vi "Module - License.vi"(8 "Error In":errorcluster, 10 "License Filename":string="lcs_daq.bin", 11 "Product Name":string="VSys DAQ") -> (0 "Error Out":errorcluster, 1 "License Missing?":bool, 2 "Activate?":bool, 3 "License Info":T1={"Expired Time"="", "Computer ID"="", "Product Name"="", "Period"=0, "Activated Time"="", "License Level"=enum."Level 1", "License Type"=enum."Trial", "Log Time"=""}, 4 "Days left":i16)   [LabVIEW 2020]
doc: "This module handle the licensing part. It check the status of current license. If expired, msg will popup and ask user to activate a license or continue use as free user."
uses:
  Control/License File Parameter.ctl
  Control/State - Module License.ctl
  <vilib>/Utility/sysdir.llb/System Directory Type.ctl
panel:
  out "COMPUTER ID":string
  out "Expired?":bool
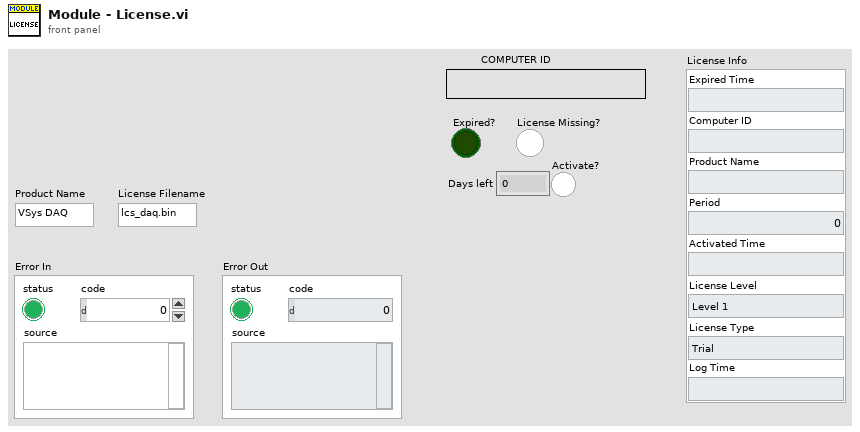
[diagram p1: front panel]
types:
  T1 = typedef "License File Parameter.ctl" = cluster{"Expired Time":string, "Computer ID":string, "Product Name":string, "Period":i16, "Activated Time":string, "License Level":enum16{"Level 1", "Level 2", "Level 3", "Level 4", "Level 5"}, "License Type":enum16{"Free", "Trial", "Subscription", "Perpetual"}, "Log Time":string}
  T2 = cluster{"T_Out":i32, "License File Param":T1, "Valid":bool, "License path":path, "Computer ID":string, "License Missing?":bool, "Path":path, "Activate?":bool, "Product Name":string, "License Filename":string, "Activation Path":path}
  T3 = typedef "State - Module License.ctl" = enum16{"Init", "Get Computer ID", "Check License File Exist?", "Copy License File", "Load License", "Check Log Time", "Check License Type", "Check License: Activated Date", "Update License: Activated Date", "Check License Period", "Update Log Time", "Check Computer ID", "Activate License: Expired", "Activate License: Trial", "Close"}
  T4 = enum16{"Free", "Trial", "Subscription", "Perpetual"}
  T5 = enum16{"Level 1", "Level 2", "Level 3", "Level 4", "Level 5"}
  T6 = enum32{"invalid app kind", "Development System", "Run Time System", "Student Edition", "Embedded LabVIEW", "Evaluation", "Custom"}
  T7 = typedef "System Directory Type.ctl" = i32
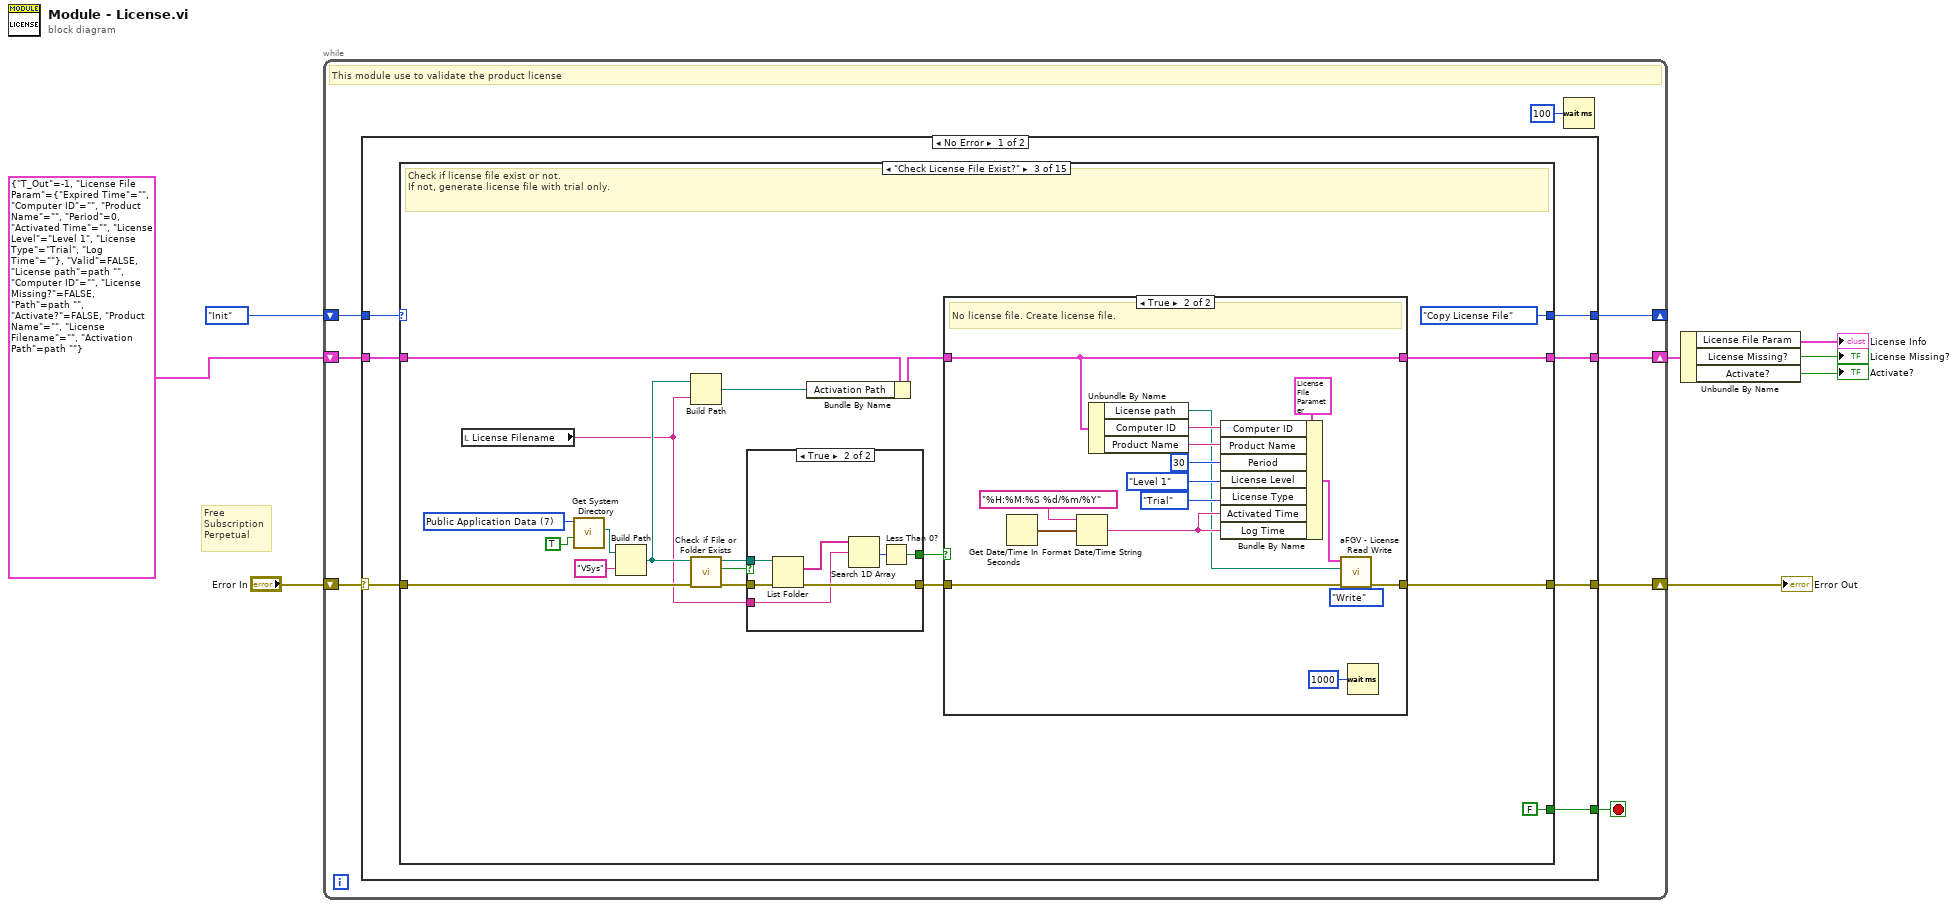
[diagram p0: block diagram]
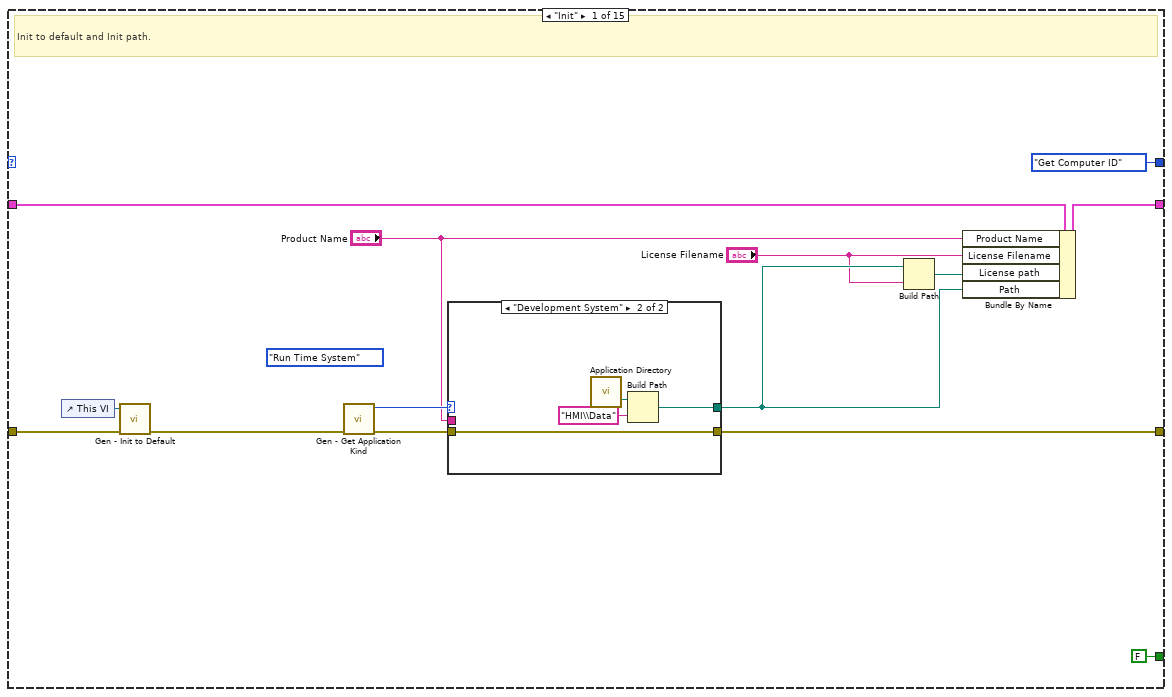
[diagram p2: hidden frame]
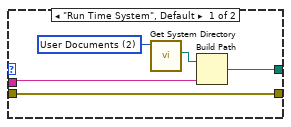
[diagram p3: hidden frame]
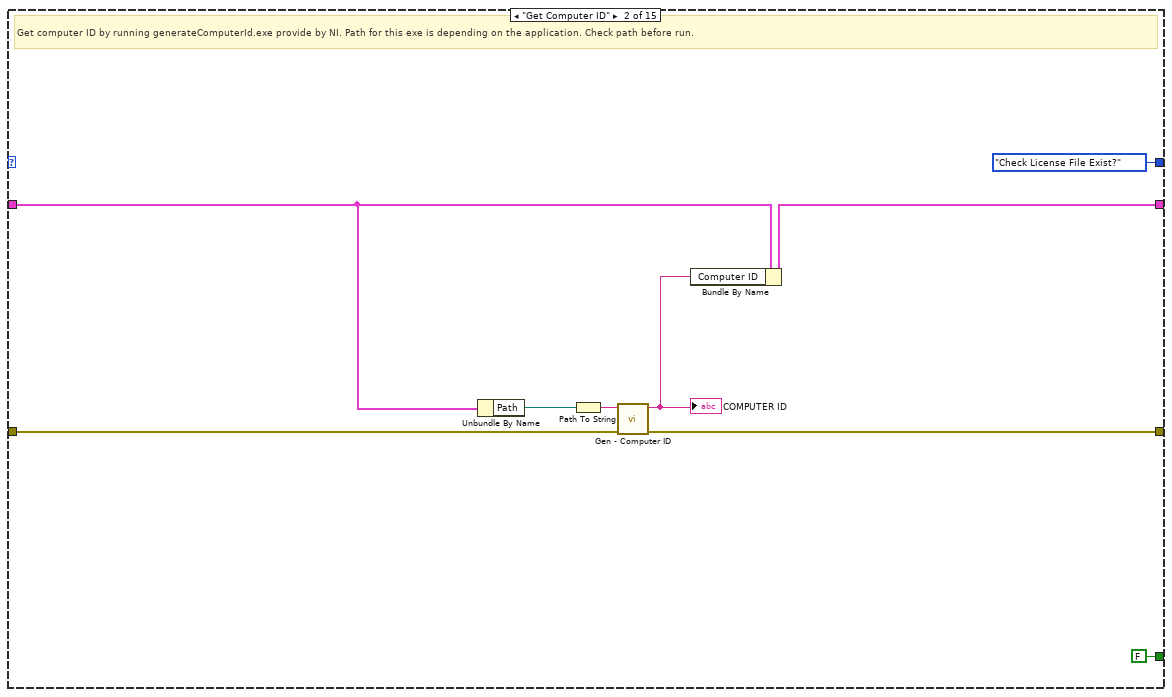
[diagram p4: hidden frame]
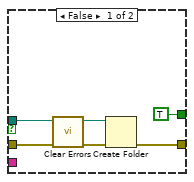
[diagram p5: hidden frame]
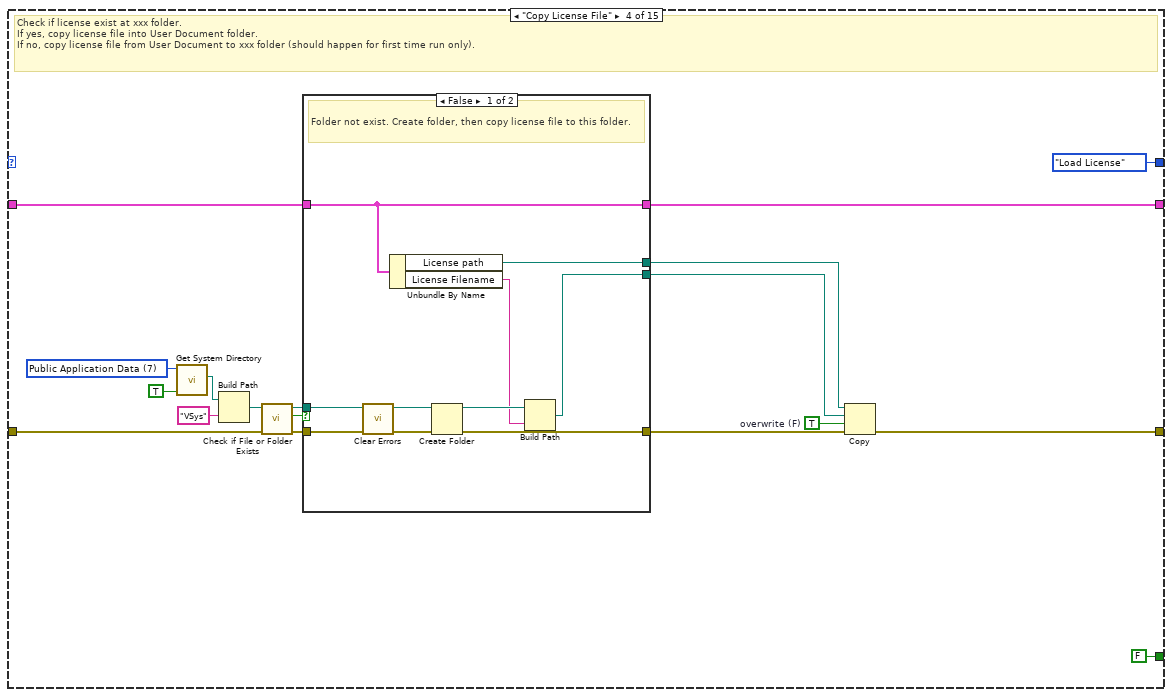
[diagram p7: hidden frame]
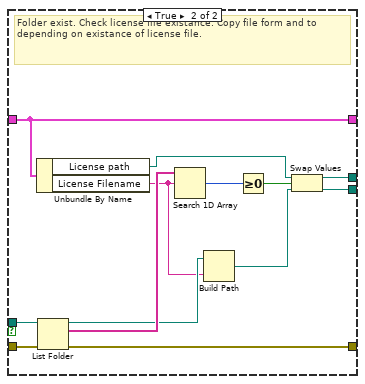
[diagram p8: hidden frame]
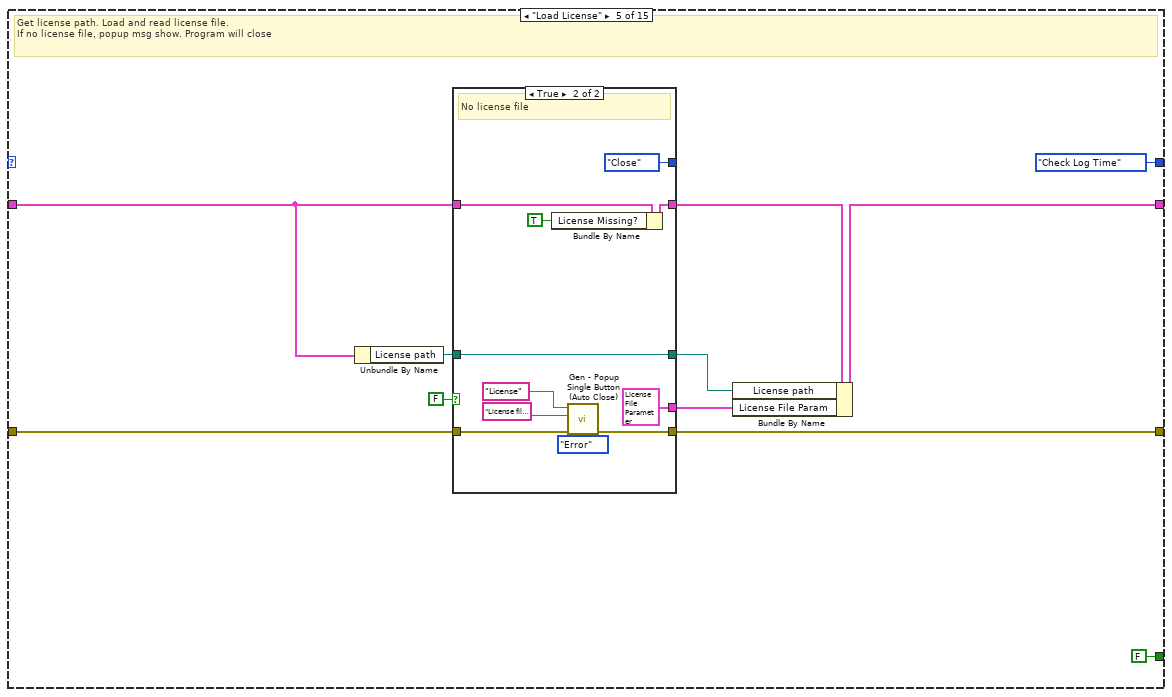
[diagram p9: hidden frame]
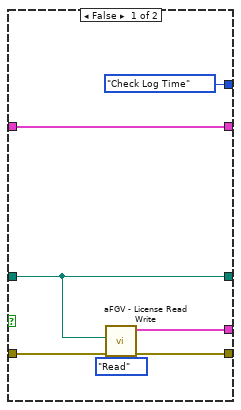
[diagram p10: hidden frame]
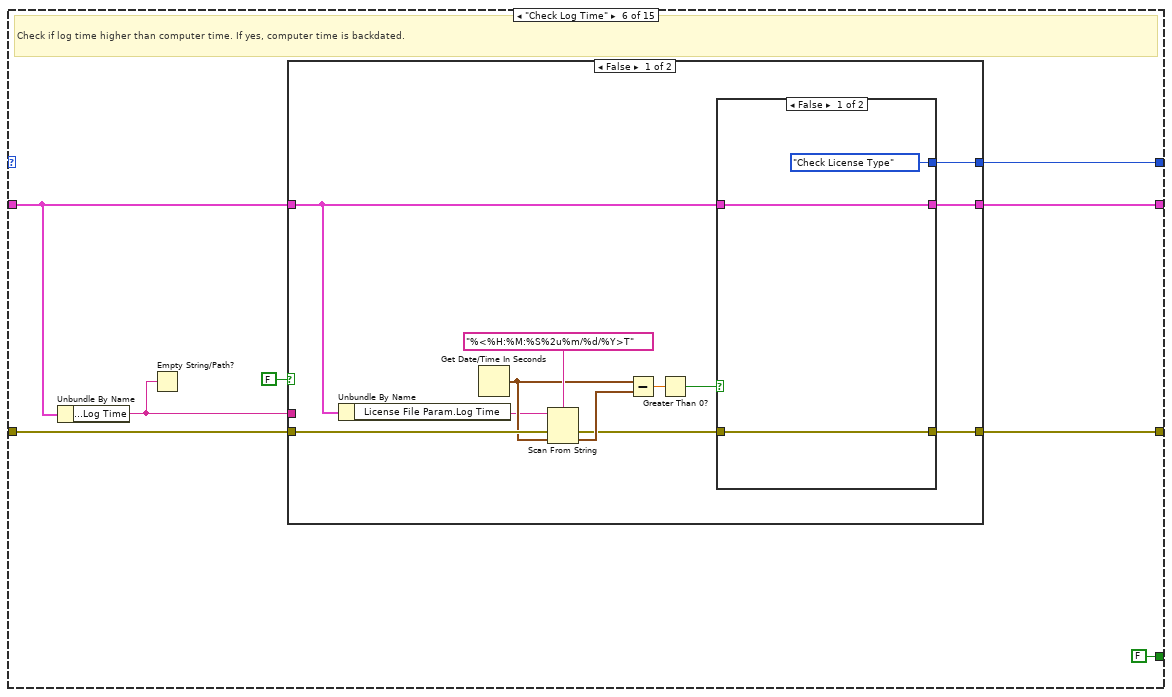
[diagram p11: hidden frame]
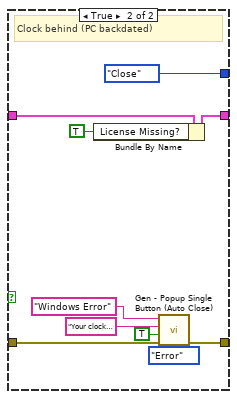
[diagram p12: hidden frame]
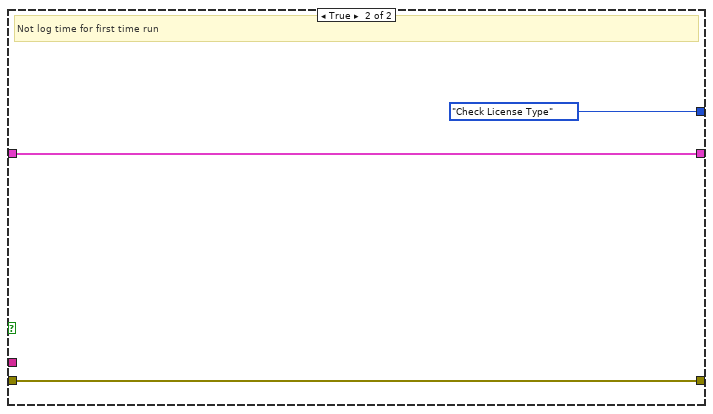
[diagram p13: hidden frame]
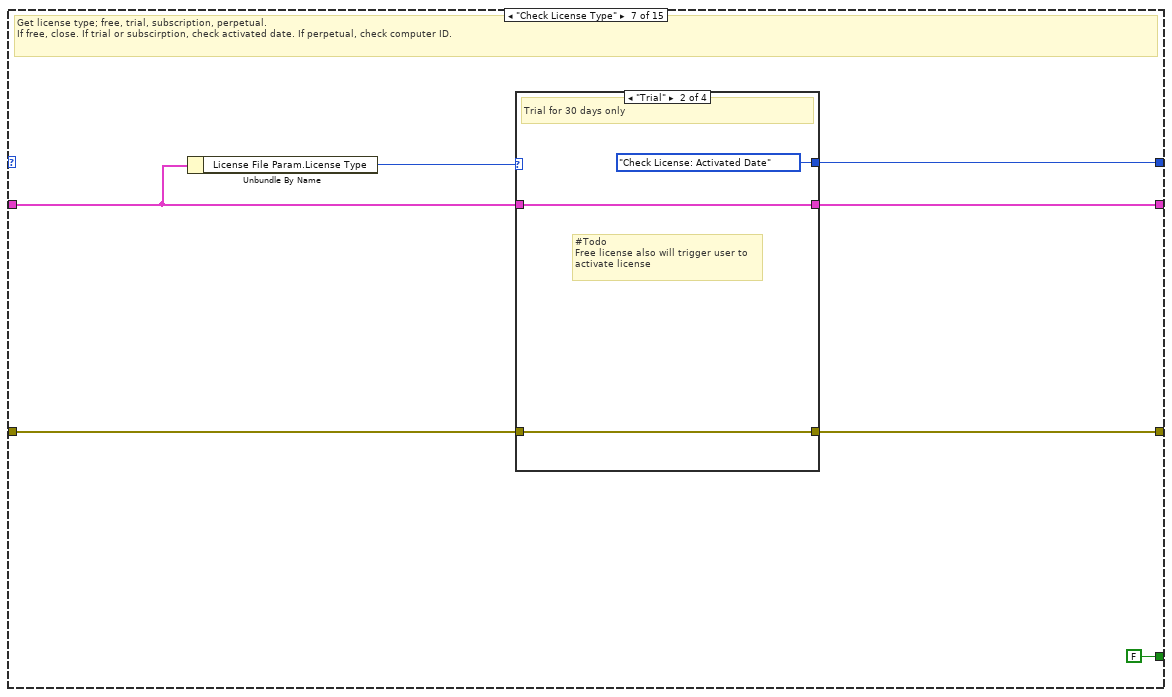
[diagram p14: hidden frame]
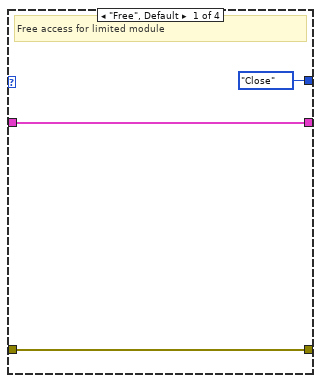
[diagram p15: hidden frame]
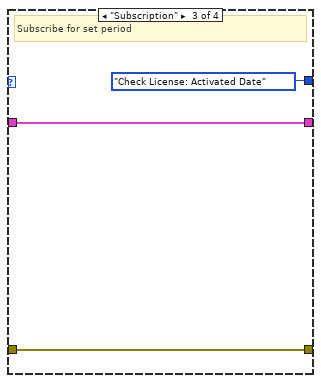
[diagram p16: hidden frame]
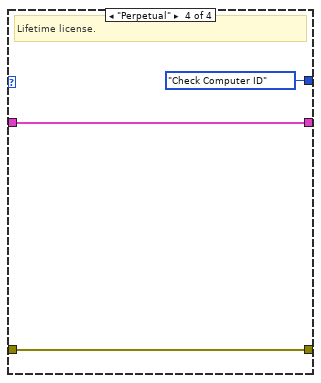
[diagram p17: hidden frame]
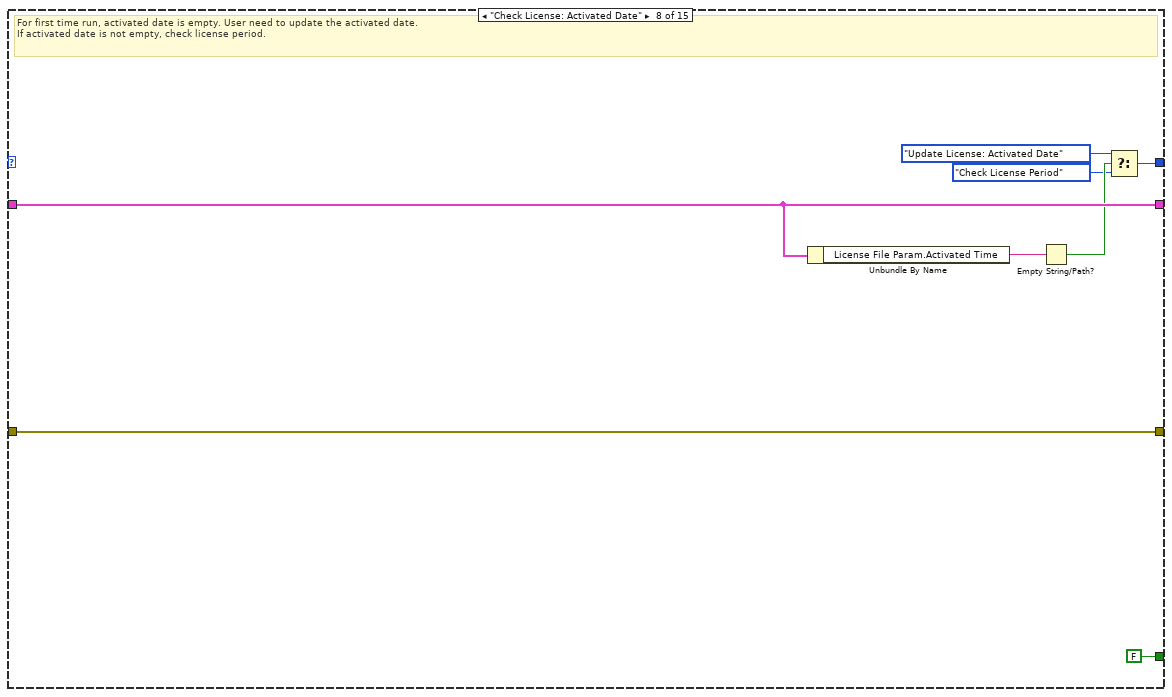
[diagram p18: hidden frame]
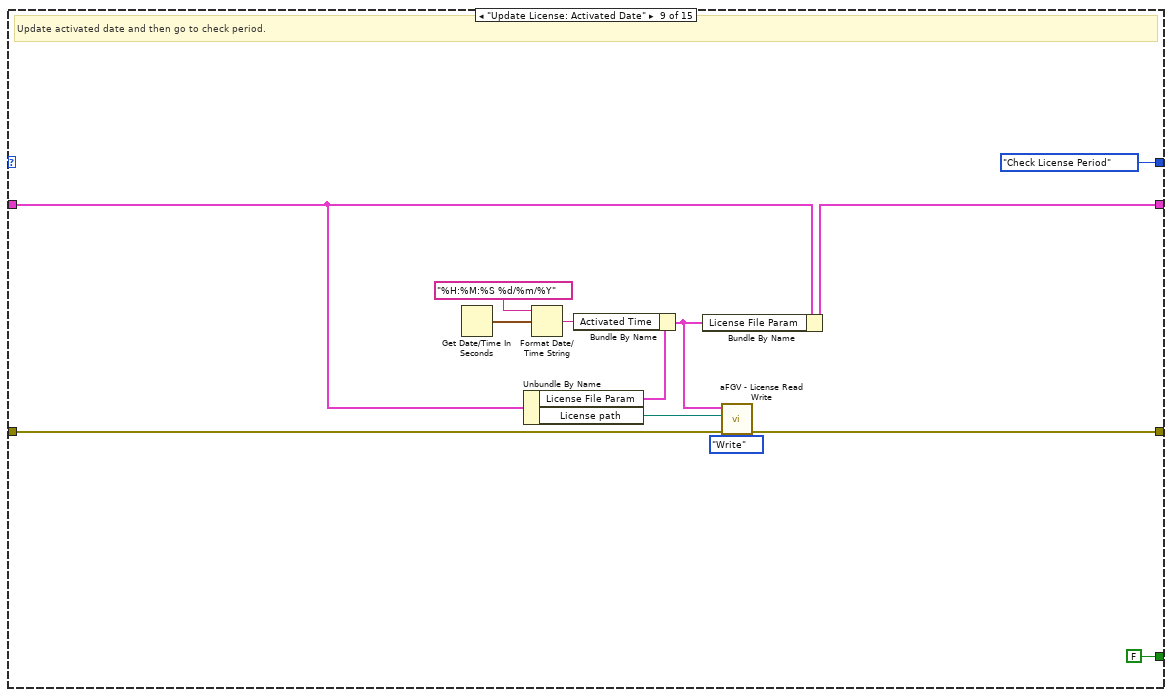
[diagram p19: hidden frame]
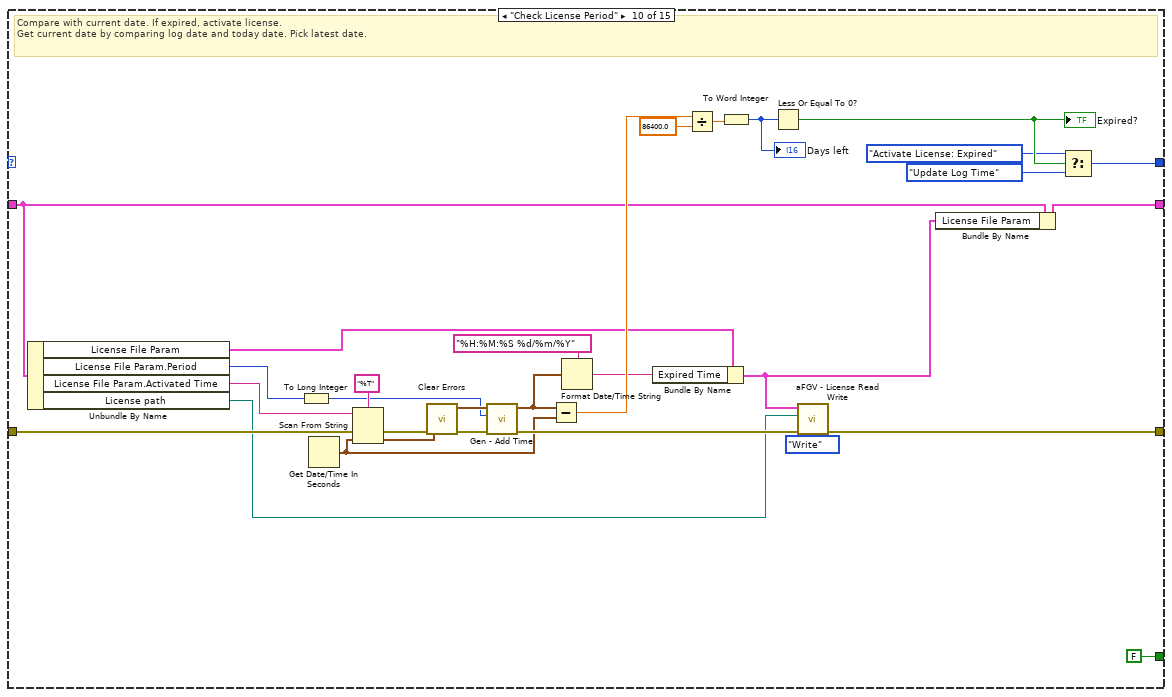
[diagram p20: hidden frame]
diagram:
  # "Free\nSubscription\nPerpetual"
  n1 = while {
    shift-right: [w12] -> _
    shift-left: State_-_Module_License."Init" -> [w14]
    shift-right: [w15] -> w7
    shift-left: "Error In" -> [w16]
    shift-right: [w9] -> w3
    shift-left: T2 {"T_Out"=-1, "License File Param"={"Expired Time"="", "Computer ID"="", "Product Name"="", "Period"=0, "Activated Time"="", "License Level"=enum."Level 1", "License Type"=enum."Trial", "Log Time"=""}, "Valid"=FALSE, "License path"=path "", "Computer ID"="", "License Missing?"=FALSE, "Path"=path "", "Activate?"=FALSE, "Product Name"="", "License Filename"="", "Activation Path"=path ""} -> [w11]
    stop <- w13 stop-if-true
    # "This module use to validate the product license"
    n2 = case shown="No Error" w16 {
      selector: w16 -> [w22 w375]
      tunnel: w14 -> [w21 w373]
      tunnel: [w23 w371] -> w15
      tunnel: [w20 TRUE] -> w13
      tunnel: [w19 w373] -> w12
      tunnel: w11 -> [w18 w372]
      tunnel: [w17 w372] -> w9
      frame No Error {
        n3 = case shown="\"Check License File Exist?\"" w21 {
          tunnel: [w31 w53 w71 w116 w153 w180 w215 w234 w246 w263 w284 w293 w322 w348 w370] -> w23
          tunnel: w22 -> [w37 w49 w63 w113 w154 w179 w214 w234 w242 w269 w285 w292 w324 w350 w370]
          tunnel: [FALSE FALSE FALSE FALSE FALSE FALSE FALSE FALSE FALSE FALSE FALSE FALSE FALSE FALSE TRUE] -> w20
          tunnel: [State_-_Module_License."Get Computer ID" State_-_Module_License."Check License File Exist?" State_-_Module_License."Copy License File" State_-_Module_License."Load License" State_-_Module_License."Check Log Time" w177 w213 w231 State_-_Module_License."Check License Period" ("f") w250 State_-_Module_License."Check Computer ID" w296 w315 State_-_Module_License."Close" State_-_Module_License."Close"] -> w19
          tunnel: w18 -> [w36 w48 w68 w108 w147 w176 w211 w235 w248 w262 w288 w295 w320 w346 w369]
          tunnel: [w32 w51 w69 w107 w152 w175 w212 w235 w244 w254 w283 w294 w319 w345 w369] -> w17
          frame "Init" {
            (unwired) T6."Run Time System" ("Application:Kind")
            # "Init to default and Init path."
            n4 = control-ref of="This VI"() -> (w34:refnum<vi>)
            n5 = call "Gen - Init to Default.vi"("Error in"=w37, "This VI"=w34) -> ("Error out"=w30:errorcluster)  [unwired: 8 in, 1 out]
            n6 = call "Gen - Get Application Kind.vi"("Error In"=w30) -> ("Error Out"=w29:errorcluster, "Application:Kind"=w25:T6)  [unwired: 9 in]
            n7 = case shown="\"Development System\"" w25 {
              tunnel: [w39 w43] -> w27
              tunnel: [w42 w46] -> w31
              tunnel: w29 -> [w42 w46]
              tunnel: "Product Name" -> [w38 _]
              frame "Run Time System", Default {
                w40 = T7 2 items=["User Home"=0, "User Desktop"=1, "User Documents"=2, "User Application Data"=3, "User Preferences"=4, "User Temporary"=5, "Public Documents"=6, "Public Application Data"=7, "Public Preferences"=8, "Public Cache"=13, "System Core Libraries"=9, "System Installed Libraries"=10, "Application Files"=11, "Boot Volume Root"=12] ("system directory type")
                n8 = call <vilib>:"Get System Directory.vi"("system directory type"=w40) -> ("system directory"=w41:path)  [unwired: 10 in]
                n9 = Build Path(base path=w41, name or relative path=w38) -> (appended path=w39:path)
              }
              frame "Development System" {
                n10 = call <vilib>:"Application Directory.vi"() -> ("Application Directory"=w44:path)
                n11 = Build Path(base path=w44, name or relative path="HMI\\Data") -> (appended path=w43:path)
              }
            }
            n12 = Build Path(base path=w27, name or relative path="License Filename") -> (appended path=w28:path)
            n13 = Bundle By Name(cluster=w36, "Product Name"="Product Name", "License Filename"="License Filename", "License path"=w28, "Path"=w27) -> (w32:T2)
          }
          frame "Get Computer ID" {
            # "Get computer ID by running generateComputerId.exe provide by NI. Path for this exe is depending on the application. Check path before run."
            n14 = Unbundle By Name(w48) -> ("Path"=w47:path)
            n15 = Path To String(path=w47) -> (string=w52:string)
            n16 = call "Gen - Computer ID.vi"("Error In"=w49, "Path"=w52) -> ("Error Out"=w53:errorcluster, "COMPUTER ID"=w50:string)  [unwired: 8 in]
            "COMPUTER ID" <- w50
            n17 = Bundle By Name(cluster=w48, "Computer ID"=w50) -> (w51:T2)
          }
          frame "Check License File Exist?" {
            w64 = T7 7 items=["User Home"=0, "User Desktop"=1, "User Documents"=2, "User Application Data"=3, "User Preferences"=4, "User Temporary"=5, "Public Documents"=6, "Public Application Data"=7, "Public Preferences"=8, "Public Cache"=13, "System Core Libraries"=9, "System Installed Libraries"=10, "Application Files"=11, "Boot Volume Root"=12] ("system directory type")
            # "Check if license file exist or not.\nIf not, generate license file with trial only."
            n18 = local read "License Filename"() -> (w56:string)
            n19 = call <vilib>:"Get System Directory.vi"("create directory if not found? (F)"=TRUE, "system directory type"=w64) -> ("system directory"=w67:path)  [unwired: 9 in]
            n20 = Build Path(base path=w67, name or relative path="VSys") -> (appended path=w58:path)
            n21 = Build Path(base path=w58, name or relative path=w56) -> (appended path=w57:path)
            n22 = call <vilib>:"Check if File or Folder Exists.vi"("error in (no error)"=w63, "path"=w58) -> ("error out"=w61:errorcluster, "file or folder exists?"=w60:bool, "dup path"=w62:path)  [unwired: 7 in]
            n23 = case shown="True" w60 {
              tunnel: [TRUE w84] -> w72
              tunnel: [w77 w83] -> w70
              tunnel: w62 -> [w78 w82]
              tunnel: w61 -> [w76 w81]
              tunnel: w56 -> [_ w80]
              frame False {
                n24 = call <vilib>:"Clear Errors.vi"("error in (no error)"=w76) -> ("error out"=w75:errorcluster)  [unwired: 5 in, 1 out]
                n25 = Create Folder(path (use dialog)=w78, error in=w75) -> (error out=w77:errorcluster)  [unwired: 1 in, 2 out]
              }
              frame True {
                n26 = List Folder(path=w82, error in=w81) -> (filenames=w86:string[], error out=w83:errorcluster)  [unwired: 2 in, 2 out]
                n27 = Search 1D Array(1D array=w86, element=w80) -> (index of element=w85:i32)  [unwired: 1 in]
                n28 = Less Than 0?(x=w85) -> (x < 0?=w84:bool)
              }
            }
            n29 = Bundle By Name(cluster=w68, "Activation Path"=w57) -> (w59:T2)
            n30 = case shown="True" w72 {
              tunnel: [w88 w103] -> w71
              tunnel: w70 -> [w88 w104]
              tunnel: [w87 w99] -> w69
              tunnel: w59 -> [w87 w99]
              frame False {
                # "License file Exist"
              }
              frame True {
                # "No license file. Create license file."
                n31 = Get Date/Time In Seconds() -> (seconds since 1Jan1904=w97:timestamp)
                n32 = Format Date/Time String(time format string (%c)="%H:%M:%S %d/%m/%Y", seconds (now)=w97) -> (date/time string=w94:string)  [unwired: 1 in]
                n33 = Unbundle By Name(w99) -> ("License path"=w90:path, "Computer ID"=w98:string, "Product Name"=w95:string)
                n34 = Bundle By Name(cluster=T1 {"Expired Time"="", "Computer ID"="", "Product Name"="", "Period"=0, "Activated Time"="", "License Level"=enum."Level 1", "License Type"=enum."Trial", "Log Time"=""} ("Data In"), "Computer ID"=w98, "Product Name"=w95, "Period"=i16 30, "License Level"=T5."Level 1", "License Type"=T4."Trial", "Activated Time"=w94, "Log Time"=w94) -> (w100:T1)
                n35 = call "aFGV - License Read Write.vi"("State"=enum16{"Read", "Write"}."Write", "Error In"=w104, "Path"=w90, "Data In"=w100) -> ("Error Out"=w103:errorcluster)  [unwired: 6 in, 1 out]
                n36 = Wait (ms)(milliseconds to wait=u32 1000) -> ()  [unwired: 1 out]
              }
            }
          }
          frame "Copy License File" {
            w115 = TRUE  # overwrite (F)
            w120 = T7 7 items=["User Home"=0, "User Desktop"=1, "User Documents"=2, "User Application Data"=3, "User Preferences"=4, "User Temporary"=5, "Public Documents"=6, "Public Application Data"=7, "Public Preferences"=8, "Public Cache"=13, "System Core Libraries"=9, "System Installed Libraries"=10, "Application Files"=11, "Boot Volume Root"=12] ("system directory type")
            # "Check if license exist at xxx folder. \nIf yes, copy license file into User Document folder.\nIf no, copy license file from User Document to xxx folder (should happen for first time run only)."
            n37 = call <vilib>:"Get System Directory.vi"("create directory if not found? (F)"=TRUE, "system directory type"=w120) -> ("system directory"=w119:path)  [unwired: 9 in]
            n38 = Build Path(base path=w119, name or relative path="VSys") -> (appended path=w111:path)
            n39 = call <vilib>:"Check if File or Folder Exists.vi"("error in (no error)"=w113, "path"=w111) -> ("error out"=w112:errorcluster, "file or folder exists?"=w109:bool, "dup path"=w110:path)  [unwired: 7 in]
            n40 = case shown="False" w109 {
              tunnel: [w130 w144] -> w114
              tunnel: w112 -> [w131 w143]
              tunnel: w110 -> [w129 w142]
              tunnel: w108 -> [w128 w141]
              tunnel: [w128 w141] -> w107
              tunnel: [w127 w133] -> w106
              tunnel: [w124 w132] -> w105
              frame False {
                # "Folder not exist. Create folder, then copy license file to this folder."
                n41 = call <vilib>:"Clear Errors.vi"("error in (no error)"=w131) -> ("error out"=w123:errorcluster)  [unwired: 5 in, 1 out]
                n42 = Unbundle By Name(w128) -> ("License path"=w127:path, "License Filename"=w125:string)
                n43 = Create Folder(path (use dialog)=w129, error in=w123) -> (created path=w126:path, error out=w130:errorcluster)  [unwired: 1 in, 1 out]
                n44 = Build Path(base path=w126, name or relative path=w125) -> (appended path=w124:path)
              }
              frame True {
                # "Folder exist. Check license file existance. Copy file form and to depending on existance of license file."
                n45 = Unbundle By Name(w141) -> ("License path"=w135:path, "License Filename"=w137:string)
                n46 = List Folder(path=w142, error in=w143) -> (path out=w138:path, filenames=w140:string[], error out=w144:errorcluster)  [unwired: 2 in, 1 out]
                n47 = Search 1D Array(1D array=w140, element=w137) -> (index of element=w139:i32)  [unwired: 1 in]
                n48 = Build Path(base path=w138, name or relative path=w137) -> (appended path=w134:path)
                n49 = Greater Or Equal To 0?(x=w139) -> (x >= 0?=w136:bool)
                n50 = Swap Values(12:w135, 13:w136, 14:w134) -> (1:w133:path, 3:w132:path)
              }
            }
            n51 = Copy(8:w114, 9:w115, 10:w105, 11:w106) -> (0:w116:errorcluster)  [unwired: 1 in, 2 out]
          }
          frame "Load License" {
            # "Get license path. Load and read license file. \nIf no license file, popup msg show. Program will close"
            n52 = Unbundle By Name(w147) -> ("License path"=w146:path)
            n53 = case shown="True" FALSE {
              tunnel: w154 -> [w162 w172]
              tunnel: [w161 w171] -> w153
              tunnel: w146 -> [w157 w167]
              tunnel: [w159 T1 {"Expired Time"="", "Computer ID"="", "Product Name"="", "Period"=0, "Activated Time"="", "License Level"=enum."Level 3", "License Type"=enum."Free", "Log Time"=""} ("Data Out")] -> w151
              tunnel: [State_-_Module_License."Check Log Time" State_-_Module_License."Close"] -> _
              tunnel: [w157 w167] -> w150
              tunnel: [w156 w164] -> w149
              tunnel: w147 -> [w156 w165]
              frame False {
                n54 = call "aFGV - License Read Write.vi"("State"=enum16{"Read", "Write"}."Read", "Error In"=w162, "Path"=w157) -> ("Error Out"=w161:errorcluster, "Data Out"=w159:T1)  [unwired: 7 in]
              }
              frame True {
                # "No license file"
                n55 = Bundle By Name(cluster=w165, "License Missing?"=TRUE) -> (w164:T2)
                n56 = call "Gen - Popup Single Button (Auto Close).vi"("Type"=enum16{"Error", "Info"}."Error", "Error in"=w172, "Message in"="License file not found. \nProgram will close." ("Header"), "Header"="License") -> ("Error out"=w171:errorcluster)  [unwired: 6 in, 1 out]
              }
            }
            n57 = Bundle By Name(cluster=w149, "License path"=w150, "License File Param"=w151) -> (w152:T2)
          }
          frame "Check Log Time" {
            # "Check if log time higher than computer time. If yes, computer time is backdated."
            n58 = Unbundle By Name(w176) -> ("License File Param.Log Time"=w178:string)
            n59 = Empty String/Path?(string/path=w178) -> ()  [unwired: 1 out]
            n60 = case shown="False" FALSE {
              tunnel: [w187 w209] -> w180
              tunnel: w179 -> [w192 w209]
              tunnel: w178 -> [_ _]
              tunnel: [w185 State_-_Module_License."Check License Type"] -> w177
              tunnel: w176 -> [w183 w207]
              tunnel: [w184 w207] -> w175
              frame False {
                n61 = Unbundle By Name(w183) -> ("License File Param.Log Time"=w182:string)
                n62 = Get Date/Time In Seconds() -> (seconds since 1Jan1904=w191:timestamp)
                n63 = Scan From String(format string="%<%H:%M:%S%2u%m/%d/%Y>T", input string=w182, error in=w192, default 1=w191) -> (error out=w188:errorcluster, output 1=w190:timestamp)  [unwired: 1 in, 2 out]
                n64 = Subtract(x=w191, y=w190) -> (x-y=w189:dbl)
                n65 = Greater Than 0?(x=w189) -> (x > 0?=w186:bool)
                n66 = case shown="False" w186 {
                  tunnel: w188 -> [w196 w204]
                  tunnel: [w196 w203] -> w187
                  tunnel: [State_-_Module_License."Check License Type" State_-_Module_License."Close"] -> w185
                  tunnel: [w194 w199] -> w184
                  tunnel: w183 -> [w194 w200]
                  frame False {
                  }
                  frame True {
                    # "Clock behind (PC backdated)"
                    n67 = Bundle By Name(cluster=w200, "License Missing?"=TRUE) -> (w199:T2)
                    n68 = call "Gen - Popup Single Button (Auto Close).vi"("Type"=enum16{"Error", "Info"}."Error", "Error in"=w204, "Auto Close? F"=TRUE, "Message in"="Your clock is behind.\n\nCannot load software program because the date and time are incorrect." ("Header"), "Header"="Windows Error") -> ("Error out"=w203:errorcluster)  [unwired: 5 in, 1 out]
                  }
                }
              }
              frame True {
                # "Not log time for first time run"
              }
            }
          }
          frame "Check License Type" {
            # "Get license type; free, trial, subscription, perpetual.\nIf free, close. If trial or subscirption, check activated date. If perpetual, check computer ID."
            n69 = Unbundle By Name(w211) -> ("License File Param.License Type"=w210:T4)
            n70 = case shown="\"Trial\"" w210 {
              tunnel: [w219 w222 w225 w228] -> w215
              tunnel: w214 -> [w219 w222 w225 w228]
              tunnel: [State_-_Module_License."Close" State_-_Module_License."Check License: Activated Date" State_-_Module_License."Check License: Activated Date" State_-_Module_License."Check Computer ID"] -> w213
              tunnel: [w217 w220 w223 w226] -> w212
              tunnel: w211 -> [w217 w220 w223 w226]
              frame "Free", Default {
                # "Free access for limited module"
              }
              frame "Trial" {
                # "#Todo\nFree license also will trigger user to \nactivate license"
                # "Trial for 30 days only"
              }
              frame "Subscription" {
                # "Subscribe for set period"
              }
              frame "Perpetual" {
                # "Lifetime license."
              }
            }
          }
          frame "Check License: Activated Date" {
            # "For first time run, activated date is empty. User need to update the activated date.\nIf activated date is not empty, check license period."
            n71 = Unbundle By Name(w235) -> ("License File Param.Activated Time"=w233:string)
            n72 = Empty String/Path?(string/path=w233) -> (empty?=w232:bool)
            n73 = Select(t=State_-_Module_License."Update License: Activated Date", s=w232, f=State_-_Module_License."Check License Period") -> (s? t:f=w231:T3)
          }
          frame "Update License: Activated Date" {
            # "Update activated date and then go to check period."
            n74 = Get Date/Time In Seconds() -> (seconds since 1Jan1904=w240:timestamp)
            n75 = Unbundle By Name(w248) -> ("License File Param"=w241:T1, "License path"=w237:path)
            n76 = Format Date/Time String(time format string (%c)="%H:%M:%S %d/%m/%Y", seconds (now)=w240) -> (date/time string=w239:string)  [unwired: 1 in]
            n77 = Bundle By Name(cluster=w241, "Activated Time"=w239) -> (w243:T1)
            n78 = Bundle By Name(cluster=w248, "License File Param"=w243) -> (w244:T2)
            n79 = call "aFGV - License Read Write.vi"("State"=enum16{"Read", "Write"}."Write", "Error In"=w242, "Path"=w237, "Data In"=w243) -> ("Error Out"=w246:errorcluster)  [unwired: 6 in, 1 out]
          }
          frame "Check License Period" {
            # "Compare with current date. If expired, activate license.\nGet current date by comparing log date and today date. Pick latest date."
            n80 = Unbundle By Name(w262) -> ("License File Param"=w255:T1, "License File Param.Period"=w272:i16, "License File Param.Activated Time"=w265:string, "License path"=w256:path)
            n81 = To Long Integer(number=w272) -> (32bit integer=w266:i32)
            n82 = Get Date/Time In Seconds() -> (seconds since 1Jan1904=w260:timestamp)
            n83 = Scan From String(format string="%T", input string=w265, error in=w269, default 1=w260) -> (error out=w268:errorcluster, output 1=w271:timestamp)  [unwired: 1 in, 2 out]
            n84 = call <vilib>:"Clear Errors.vi"("error in (no error)"=w268) -> ("error out"=w267:errorcluster)  [unwired: 5 in, 1 out]
            n85 = call "Gen - Add Time.vi"("Error In"=w267, "#days"=w266, "Time In"=w271) -> ("Error Out"=w264:errorcluster, "Time Out"=w259:timestamp)  [unwired: 7 in]
            n86 = Subtract(x=w259, y=w260) -> (x-y=w270:dbl)
            n87 = Format Date/Time String(time format string (%c)="%H:%M:%S %d/%m/%Y", seconds (now)=w259) -> (date/time string=w258:string)  [unwired: 1 in]
            n88 = Bundle By Name(cluster=w255, "Expired Time"=w258) -> (w253:T1)
            n89 = Divide(x=w270, y=86400.0) -> (x/y=w276:dbl)
            n90 = To Word Integer(number=w276) -> (16bit integer=w277:i16)
            "Days left" <- w277
            n91 = Less Or Equal To 0?(x=w277) -> (x <= 0?=w252:bool)
            "Expired?" <- w252
            n92 = call "aFGV - License Read Write.vi"("State"=enum16{"Read", "Write"}."Write", "Error In"=w264, "Path"=w256, "Data In"=w253) -> ("Error Out"=w263:errorcluster)  [unwired: 6 in, 1 out]
            n93 = Bundle By Name(cluster=w262, "License File Param"=w253) -> (w254:T2)
            n94 = Select(t=State_-_Module_License."Activate License: Expired" ("f"), s=w252, f=State_-_Module_License."Update Log Time") -> (s? t:f=w250:T3)
          }
          frame "Update Log Time" {
            n95 = Unbundle By Name(w288) -> ("License File Param"=w287:T1, "License path"=w286:path)
            n96 = Get Date/Time In Seconds() -> (seconds since 1Jan1904=w280:timestamp)
            n97 = Format Date/Time String(time format string (%c)="%H:%M:%S %d/%m/%Y", seconds (now)=w280) -> (date/time string=w279:string)  [unwired: 1 in]
            n98 = Bundle By Name(cluster=w287, "Log Time"=w279) -> (w282:T1)
            n99 = call "aFGV - License Read Write.vi"("State"=enum16{"Read", "Write"}."Write", "Error In"=w285, "Path"=w286, "Data In"=w282) -> ("Error Out"=w284:errorcluster)  [unwired: 6 in, 1 out]
            n100 = Bundle By Name(cluster=w288, "License File Param"=w282) -> (w283:T2)
          }
          frame "Check Computer ID" {
            # "Compare computer ID."
            n101 = Unbundle By Name(w295) -> ("Computer ID"=w298:string, "License File Param.Computer ID"=w299:string)
            n102 = Equal?(x=w298, y=w299) -> (x = y?=w297:bool)
            n103 = case shown="False" w297 {
              tunnel: [State_-_Module_License."Activate License: Expired" w306] -> w296
              tunnel: [w304 w312] -> w294
              tunnel: w295 -> [w303 w312]
              tunnel: [w301 w313] -> w293
              tunnel: w292 -> [w301 w313]
              frame False {
                n104 = Unbundle By Name(w303) -> ("Computer ID"=w302:string)
                n105 = Bundle By Name(cluster=w303, "License File Param.Computer ID"=w302) -> (w304:T2)
              }
              frame True {
                n106 = Unbundle By Name(w312) -> ("License File Param.License Type"=w311:T4)
                n107 = Equal?(x=w311, y=T4."Trial") -> (x = y?=w309:bool)
                n108 = Select(t=State_-_Module_License."Activate License: Trial", s=w309, f=State_-_Module_License."Close") -> (s? t:f=w306:T3)
              }
            }
          }
          frame "Activate License: Expired" {
            # "Request user to activate license if license expired."
            n109 = call "Gen - Popup Two Button.vi"("Type"=enum16{"Error", "Info"}."Error", "Error in"=w324, "Button text"=string[] ["ACTIVATE", "CONTINUE"], "Message in"="Your license is either invalid or expired. Please activate the license.\nClick continue to use free features.", "Header"="License Activation") -> ("Error out"=w321:errorcluster, "Yes?"=w314:bool)  [unwired: 5 in]
            n110 = case shown="True" w314 {
              tunnel: [w332 w341] -> w322
              tunnel: w321 -> [w332 w342]
              tunnel: [w331 w339] -> w319
              tunnel: w320 -> [w333 w340]
              tunnel: [FALSE ("Cancel?") w338] -> w318
              frame False {
                # "Continue as free user. Level 3.\nCheck the features of each Level before define."
                n111 = Bundle By Name(cluster=w333, "License File Param.License Level"=T5."Level 3") -> (w331:T2)
              }
              frame True {
                # "Activate License. Cancel = F is user license activation success."
                n112 = Unbundle By Name(w340) -> ("License File Param"=w337:T1, "Activation Path"=w336:path, "Product Name"=w334:string)
                n113 = call "Gen - License Activator.vi"("Error In"=w342, "Product Name"=w334, "License Path"=w336, "License Param"=w337) -> ("Error Out"=w341:errorcluster, "Cancel?"=w338:bool, "Updated License Param"=w335:T1)  [unwired: 5 in]
                n114 = Bundle By Name(cluster=w340, "License File Param"=w335) -> (w339:T2)
              }
            }
            n115 = Select(t=State_-_Module_License."Activate License: Expired", s=w318, f=State_-_Module_License."Close") -> (s? t:f=w315:T3)
          }
          frame "Activate License: Trial" {
            # "Request user to activate license if license expired."
            n116 = call "Gen - Popup Two Button.vi"("Type"=enum16{"Error", "Info"}."Error", "Error in"=w350, "Button text"=string[] ["ACTIVATE", "CONTINUE"], "Message in"="You are using VSys DAQ trial version. Please activate the license.\nClick continue to keep using trial version. ", "Header"="License Activation") -> ("Error out"=w347:errorcluster, "Yes?"=w344:bool)  [unwired: 5 in]
            n117 = case shown="True" w344 {
              tunnel: [w355 w365] -> w348
              tunnel: w347 -> [w355 w366]
              tunnel: [w356 w363] -> w345
              tunnel: w346 -> [w356 w364]
              frame False {
                # "Continue as trial version."
              }
              frame True {
                # "Activate License. Cancel = F is user license activation success."
                n118 = Unbundle By Name(w364) -> ("License File Param"=w359:T1, "Activation Path"=w362:path, "Product Name"=w361:string)
                n119 = call "Gen - License Activator.vi"("Error In"=w366, "Product Name"=w361, "License Path"=w362, "License Param"=w359) -> ("Error Out"=w365:errorcluster, "Cancel?"=w360:bool, "Updated License Param"=w358:T1)  [unwired: 5 in]
                n120 = Select(t=w359, s=w360, f=w358) -> (s? t:f=w357:T1)
                n121 = Bundle By Name(cluster=w364, "License File Param"=w357) -> (w363:T2)
              }
            }
          }
          frame "Close" {
          }
        }
      }
      frame Error {
        n122 = call <vilib>:"Clear Errors.vi"("error in (no error)"=w375) -> ("error out"=w371:errorcluster)  [unwired: 5 in, 1 out]
      }
    }
    n123 = Wait (ms)(milliseconds to wait=u32 100) -> ()  [unwired: 1 out]
  }
  "Error Out" <- w7
  n124 = Unbundle By Name(w3) -> ("License File Param"=→"License Info":T1, "License Missing?"=→"License Missing?":bool, "Activate?"=→"Activate?":bool)
